vi "Initialize-client.vi"(8 "error in (no error)":errorcluster, 9 "Client channel":refnum<queue>, 10 "Server channel":refnum<queue>, 11 "Object ref in":T1) -> (0 "error out":errorcluster, 3 "Object ref out":T1)   [LabVIEW 2013, in "PowderDeposition.lvlib" / "PD-Main.lvclass"]
uses:
  PD-Main.lvclass
  Object-reference.ctl
  SA-SLMAPI/Sources/Message.lvclass
  PD-Main.lvclass/PD-Main.ctl
  Communication/Sources/PD-Client.lvclass
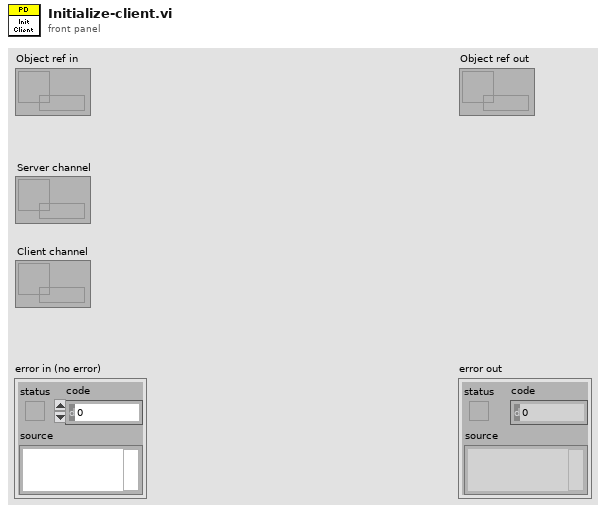
[diagram p1: front panel]
types:
  T1 = typedef "PowderDeposition.lvlib/PD-Main.lvclass/Object-reference.ctl" = refnum<data-value>
  T2 = typedef "PowderDeposition.lvlib/PD-Client.lvclass/Object-reference.ctl" = refnum<data-value>
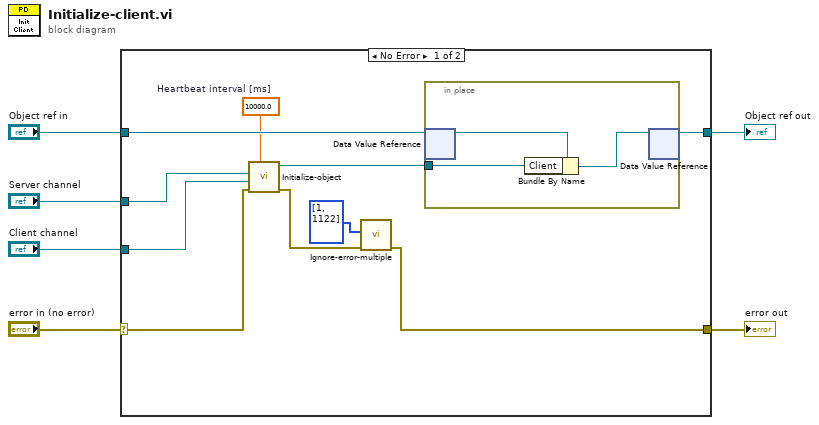
[diagram p0: block diagram]
diagram:
  n1 = case shown="No Error" "error in (no error)" {
    selector: "error in (no error)" -> [w9 w21]
    tunnel: [w8 w21] -> w5
    tunnel: [w15 w20] -> w3
    tunnel: "Object ref in" -> [w16 w20]
    tunnel: "Client channel" -> [w12 _]
    tunnel: "Server channel" -> [w13 _]
    frame No Error {
      w14 = 10000.0  # Heartbeat interval [ms]
      n2 = call "Initialize-object.vi"("Heartbeat interval"=w14, "error in (no error)"=w9, "Client channel"=w12, "Server channel"=w13) -> ("error out"=w10:errorcluster, "Reference out"=w11:T2)  [unwired: 6 in]
      n3 = call "Ignore-error-multiple.vi"("error in (no error)"=w10, "Errors to ignore (1)"=i32[] [1, 1122]) -> ("error out"=w8:errorcluster)  [unwired: 9 in]
      n4 = in-place {
        in-place-border: w11 -> [w17]
        n5 = in-place-dvr #1(w16) -> (w19:refnum<class "PD-Main.lvclass">)  [unwired: 1 out]
        n6 = Bundle By Name(cluster=w19, "Client"=w17) -> (w18:refnum<class "PD-Main.lvclass">)
        n7 = in-place-dvr #1(w18) -> (w15:T1)  [unwired: 1 out]
      }
    }
    frame Error {
    }
  }
  "error out" <- w5
  "Object ref out" <- w3
